vi "SR.vi"(7 "Spoken text box":refnum<vi>) -> (3 "event callback refnum":refnum<k27>)   [LabVIEW 2013]
uses:
  System.Speech
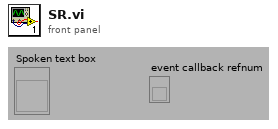
[diagram p1: front panel]
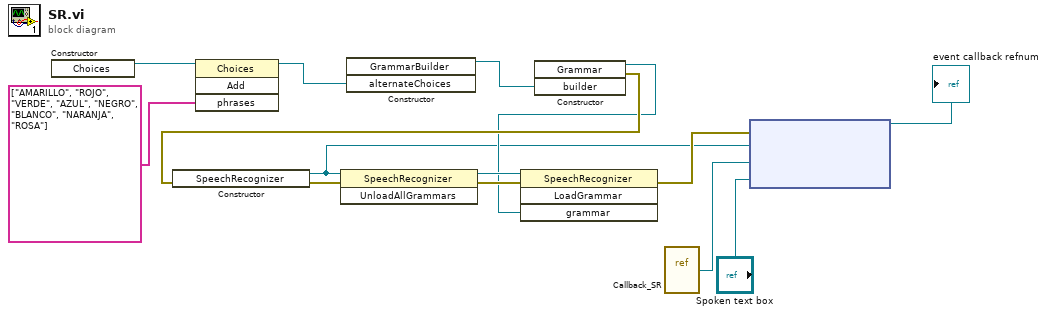
[diagram p0: block diagram]
diagram:
  n1 = constructor class="Choices"() -> (reference out=w14:refnum<k24>)  [unwired: 3 in, 2 out]
  n2 = invoke class="Choices" method="Add"(reference=w14, "phrases"=string[] ["AMARILLO", "ROJO", "VERDE", "AZUL", "NEGRO", "BLANCO", "NARANJA", "ROSA"]) -> (reference out=w12:refnum<k24>)  [unwired: 2 in, 3 out]
  n3 = constructor class="GrammarBuilder"("alternateChoices"=w12) -> (reference out=w11:refnum<k24>)  [unwired: 3 in, 3 out]
  n4 = constructor class="Grammar"("builder"=w11) -> (reference out=w6:refnum<k24>, error out=w9:errorcluster)  [unwired: 3 in, 2 out]
  n5 = constructor class="SpeechRecognizer"(error in=w9) -> (reference out=w1:refnum<k24>, error out=w10:errorcluster)  [unwired: 2 in, 1 out]
  n6 = invoke class="SpeechRecognizer" method="UnloadAllGrammars"(reference=w1, error in=w10) -> (reference out=w8:refnum<k24>, error out=w7:errorcluster)  [unwired: 1 in, 1 out]
  n7 = invoke class="SpeechRecognizer" method="LoadGrammar"(reference=w8, error in=w7, "grammar"=w6) -> (error out=w3:errorcluster)  [unwired: 1 in, 3 out]
  n8 = vi-ref "Callback_SR.vi"() -> ("vi reference"=w2:refnum<vi>)
  n9 = node(w3, w1, w2, "Spoken text box") -> (→"event callback refnum":refnum<k27>)  [unwired: 1 in, 1 out]
